vi "GetRGB.vi"(0 "ColorRGBA in":refnum<class "ColorRGBA.lvclass">, 11 "error in (no error)":errorcluster) -> (4 "ColorRGBA out":refnum<class "ColorRGBA.lvclass">, 6 "R":u8, 8 "G":u8, 10 "B":u8, 15 "error out":errorcluster)   [LabVIEW 2021, in "Picture2D.lvlib" / "ColorRGBA.lvclass"]
uses:
  ColorRGBA.lvclass
  ColorRGBA.lvclass/ColorRGBA.ctl
  ColorRGB/ColorRGB.lvclass
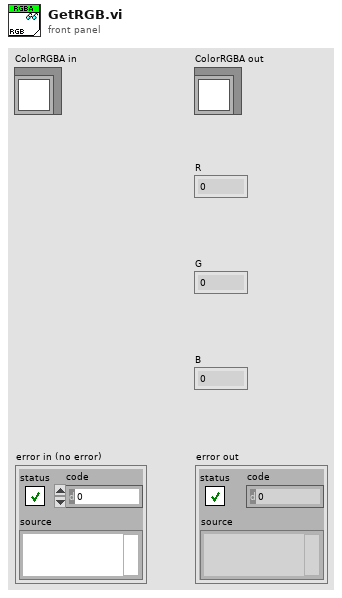
[diagram p1: front panel]
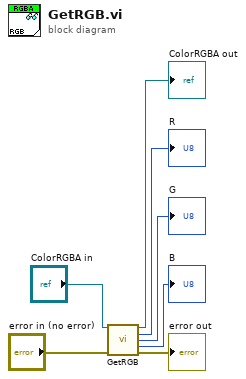
[diagram p0: block diagram]
diagram:
  n1 = call-parent "GetRGB.vi"("ColorRGB in"="ColorRGBA in", "error in (no error)"="error in (no error)") -> ("ColorRGB out"=→"ColorRGBA out":refnum<class "ColorRGBA.lvclass">, "R"=→"R":u8, "G"=→"G":u8, "B"=→"B":u8, "error out"=→"error out":errorcluster)  [unwired: 9 in]
